vi "Pipe Var Intf - Create Pipe.vi"(5 "outBufferSize (256k)":u32=256000, 7 "inBufferSize (256k)":u32=256000, 8 "error in (no error)":errorcluster, 11 "pipe name in (leave empty to generate random name)":string="\\\\.\\Pipe\\GOLPI_Variable_Pipe") -> (0 "error out":errorcluster, 2 "pipe name out":string, 3 "pipe handle out":i32)   [LabVIEW 2020, in "GOLPI library.lvlib"]
doc: "Creates named pipe of given name or random name if not provided. Creates DUPLEX pipe. Do not forget to close the handle."
uses:
  GOLPI library.lvlib
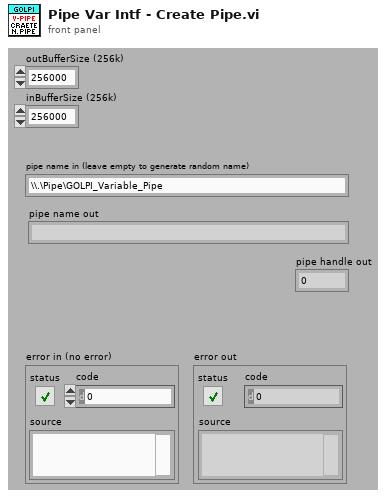
[diagram p1: front panel]
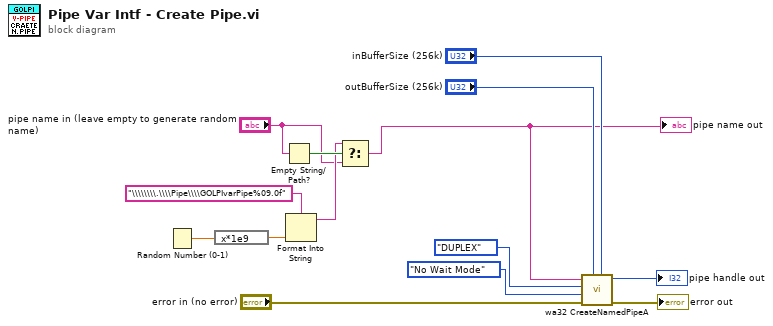
[diagram p0: block diagram]
diagram:
  n1 = Random Number (0-1)() -> (number: 0 to 1=w7:dbl)
  n2 = expression code="x*1e9"(w7) -> (w6:dbl)
  n3 = Empty String/Path?(string/path="pipe name in (leave empty to generate random name)") -> (empty?=w9:bool)
  n4 = Format Into String(format string="\\\\\\\\.\\\\Pipe\\\\GOLPIvarPipe%09.0f" ("pipe name in"), w6) -> (resulting string=w4:string)  [unwired: 2 in, 1 out]
  n5 = Select(t=w4, s=w9, f="pipe name in (leave empty to generate random name)") -> (s? t:f=w2:string)
  "pipe name out" <- w2
  n6 = call "wa32 CreateNamedPipeA.vi"("inBufferSize (256k)"="inBufferSize (256k)", "outBufferSize (256k)"="outBufferSize (256k)", "error in"="error in (no error)", "pipe mode"=enum16{"Wait Mode", "No Wait Mode"}."No Wait Mode", "open mode"=enum16{"INBOUND", "OUTBOUND", "DUPLEX"}."DUPLEX", "file path"=w2) -> ("error out"=→"error out":errorcluster, "handle"=→"pipe handle out":i32)  [unwired: 4 in]
